vi "NMT send.vi"(4 "error in (no error)":errorcluster, 5 "Node ID":u8, 6 "Command specifier":u8(ring)=1 items=["Start remote node"=1, "Stop remote node"=2, "Enter pre-operational state"=128, "Reset node"=129, "Reset communication"=130], 7 "CANopen in":refnum<class "CANopen.lvclass">) -> (0 "error out":errorcluster, 3 "CANopen out":refnum<class "CANopen.lvclass">)   [LabVIEW 2026, in "canopen_.lvlib" / "CANopen.lvclass"]
doc: "Sends a NMT message. If \"Node ID\" is not specified, the message will be broadcasted."
uses:
  CANopen.lvclass
  CANopen.lvclass/CANopen.ctl
  FunctionCode.ctl
  CANopen Master.lvlib
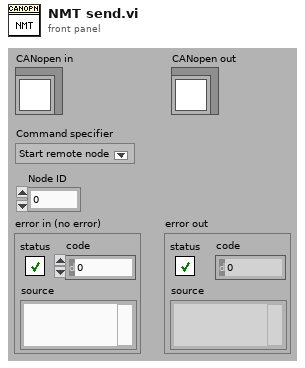
[diagram p1: front panel]
types:
  T1 = typedef "CANopen Master.lvlib/FunctionCode.ctl" = u16
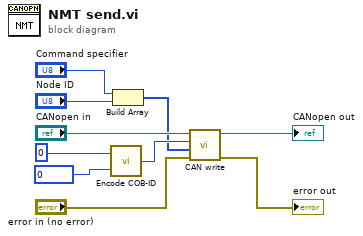
[diagram p0: block diagram]
diagram:
  w3 = T1 0 items=["EMCY"=1, "PDO1 (tx)"=3, "PDO1 (rx)"=4, "PDO2 (tx)"=5, "PDO2 (rx)"=6, "PDO3 (tx)"=7, "PDO3 (rx)"=8, "PDO4 (tx)"=9, "PDO4 (rx)"=10, "SDO (tx)"=11, "SDO (rx)"=12, "NMT error control"=14] ("Function code")
  n1 = call "Encode COB-ID.vi"("Function code"=w3, "Node-ID"=u16 0 ("Node ID")) -> ("COD-ID"=w2:u32)
  n2 = Build Array("Command specifier", "Node ID") -> (w1:u8[])
  n3 = call "CAN write.vi"("error in (no error)"="error in (no error)", "Data"=w1, "COB id"=w2, "CANopen in"="CANopen in") -> ("error out"=→"error out":errorcluster, "CANopen out"=→"CANopen out":refnum<class "CANopen.lvclass">)  [unwired: 1 in, 1 out]
